vi "tcpServerStateMachine.vi"(8 "error in (no error)":errorcluster, 9 "notifier in":refnum<notifier>, 10 "tcpServerQueue":refnum<queue>, 11 "TcpServerBase in":refnum<class "TcpServerBase.lvclass">) -> (0 "error out":errorcluster, 3 "TcpServerBase out":refnum<class "TcpServerBase.lvclass">)   [LabVIEW 2018, in "TcpServerBase.lvclass"]
doc: "TCP Server State Machine. The execution is set as Preallocated Reentrant Execution Function. This is for the two runServer.vi child functions to have two different clones.\n\nStates:\n\n1.- Create Listener.\n2.- Wait on Listener.\n3.- Read TCP Packet.\n4.- Close Connection.\n5.- Stop Server."
uses:
  TcpServerBase.lvclass
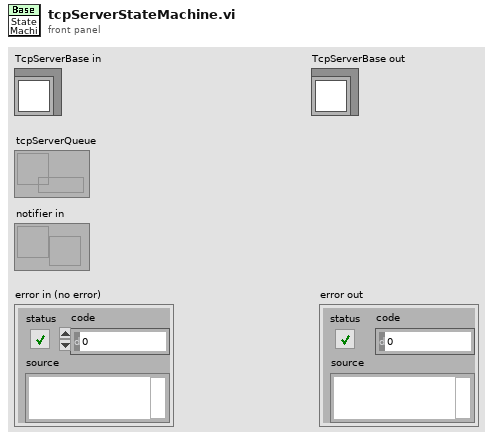
[diagram p1: front panel]
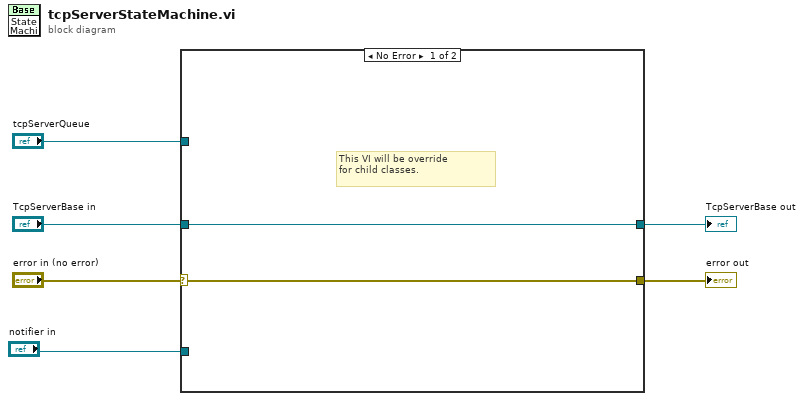
[diagram p0: block diagram]
diagram:
  n1 = case shown="No Error" "error in (no error)" {
    selector: "error in (no error)" -> [w8 w9]
    tunnel: [w8 w9] -> w5
    tunnel: [w7 w10] -> w4
    tunnel: "TcpServerBase in" -> [w7 w10]
    tunnel: "notifier in" -> [_ _]
    tunnel: "tcpServerQueue" -> [_ _]
    frame No Error {
      # "This VI will be override\nfor child classes."
    }
    frame Error {
    }
  }
  "error out" <- w5
  "TcpServerBase out" <- w4
